vi "Create.vi"(8 "Error In":errorcluster) -> (0 "Error Out":errorcluster, 3 "Compiler":refnum<class "Compiler.lvclass">)   [LabVIEW 2017, in "Mustache.lvlib" / "Compiler.lvclass"]
uses:
  Compiler.lvclass
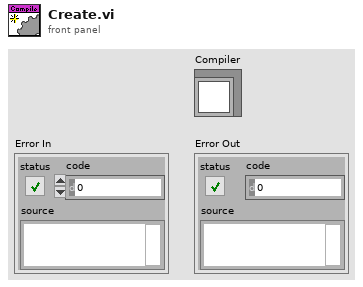
[diagram p1: front panel]
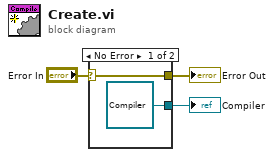
[diagram p0: block diagram]
diagram:
  n1 = case shown="No Error" "Error In" {
    selector: "Error In" -> [w5 w6]
    tunnel: [w5 w6] -> w2
    tunnel: [refnum<class "Compiler.lvclass"> refnum ("Mustache.lvlib:Compiler.lvclass") _] -> w1
    frame No Error {
    }
    frame Error {
    }
  }
  "Error Out" <- w2
  "Compiler" <- w1
